vi "test.vi"(0 "Constant (Color Operators 1)":sgl=35366.0, 1 "Color Plane (Color Plane Extraction 1)":i32(ring)=6 items=["Red", "Green", "Blue", "Hue", "Saturation", "Luminance", "Value", "Intensity"], 2 "Range (Threshold 1)":cluster{"Lower value":sgl, "Upper value":sgl}={"Lower value"=46.0, "Upper value"=97.0}, 7 "error in":errorcluster) -> (27 "error out":errorcluster)   [LabVIEW 2009]
uses:
  <vilib>/vision/NI_Vision_Development_Module.lvlib
panel:
  out "Image Out":T1(plugin-control)
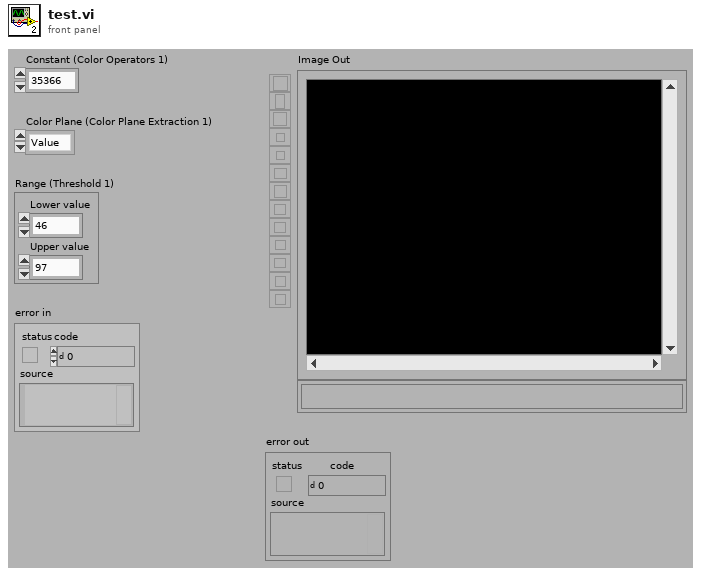
[diagram p1: front panel]
types:
  T1 = typedef "IMAQ Image.ctl" = refnum<image>
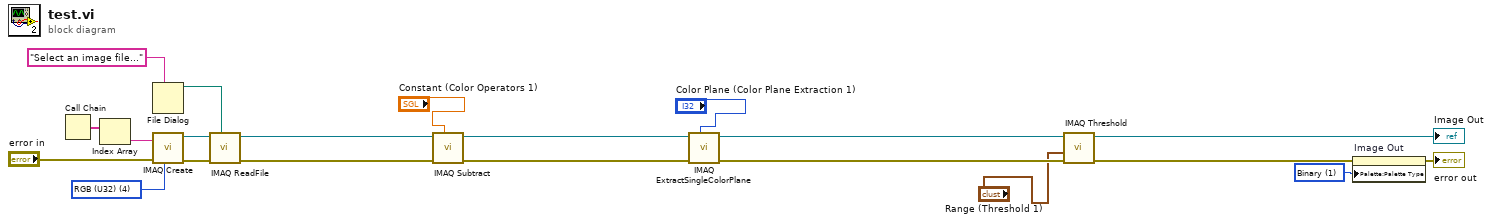
[diagram p0: block diagram]
diagram:
  w2 = u32 1 items=["Grayscale", "Binary", "Gradient", "Rainbow", "Temperature", "User Defined"] ("Palette")
  w18 = u32 4 items=["Grayscale (U8)", "Grayscale (I16)", "Grayscale (SGL)", "Complex (CSG)", "RGB (U32)", "HSL (U32)", "RGB (U64)"] ("Image Type")
  n1 = Call Chain() -> (call chain=w14:string[])
  n2 = Index Array(array=w14) -> (element=w13:string)  [unwired: 1 in]
  n3 = File Dialog(7:"Select an image file..." ("prompt")) -> (3:w17:path)  [unwired: 1 in, 8 out]
  n4 = call "IMAQ Create"("Image Name"=w13, "Image Type"=w18, "error in (no error)"="error in") -> ("New Image"=w20:T1, "error out"=w19:errorcluster)  [unwired: 1 in, 1 out]
  n5 = call "IMAQ ReadFile"("File Path"=w17, "error in (no error)"=w19, "Image"=w20) -> ("error out"=w21:errorcluster, "Image Out"=w11:T1)  [unwired: 2 in, 5 out]
  n6 = call "IMAQ Subtract"("Image Src A"=w11, "Constant"="Constant (Color Operators 1)", "error in (no error)"=w21) -> ("Image Dst Out"=w8:T1, "error out"=w10:errorcluster)  [unwired: 2 in, 2 out]
  n7 = call "IMAQ ExtractSingleColorPlane"("Color Plane"="Color Plane (Color Plane Extraction 1)", "error in (no error)"=w10, "Image Src"=w8) -> ("error out"=w7:errorcluster, "Image Dst Out"=w5:T1)  [unwired: 1 in, 6 out]
  n8 = call "IMAQ Threshold"("error in (no error)"=w7, "Range"="Range (Threshold 1)", "Image Src"=w5) -> ("error out"=w4:errorcluster, "Image Dst Out"=→"Image Out":T1)  [unwired: 3 in, 4 out]
  n9 = property on="Image Out" class="ImageControl"(error in=w4, "Palette:Palette Type"=w2) -> (error out=→"error out":errorcluster)  [unwired: 1 in, 1 out]
